vi "Load Class.vi"(8 "error in":errorcluster, 10 "PPLs Folder Path":path, 11 "Configuration in":refnum<class "Configuration.lvclass">) -> (0 "error out":errorcluster, 2 "Class out":refnum<class>, 3 "Configuration out":refnum<class "Configuration.lvclass">)   [LabVIEW 2018, in "Configuration.lvlib" / "Configuration.lvclass"]
doc: "Load the specific class and return a generic class instantiation"
uses:
  Configuration.lvclass
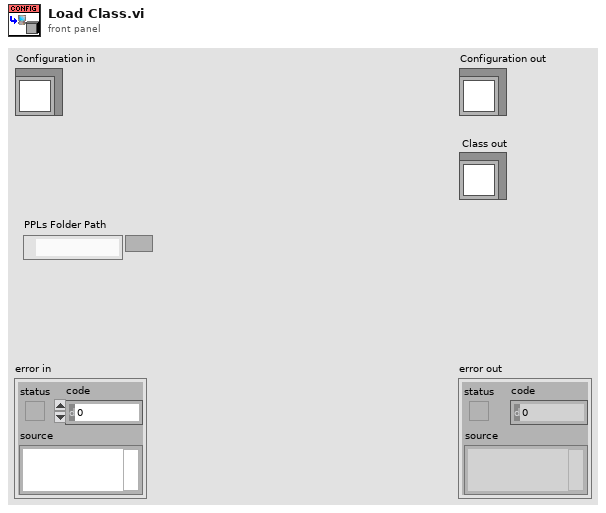
[diagram p1: front panel]
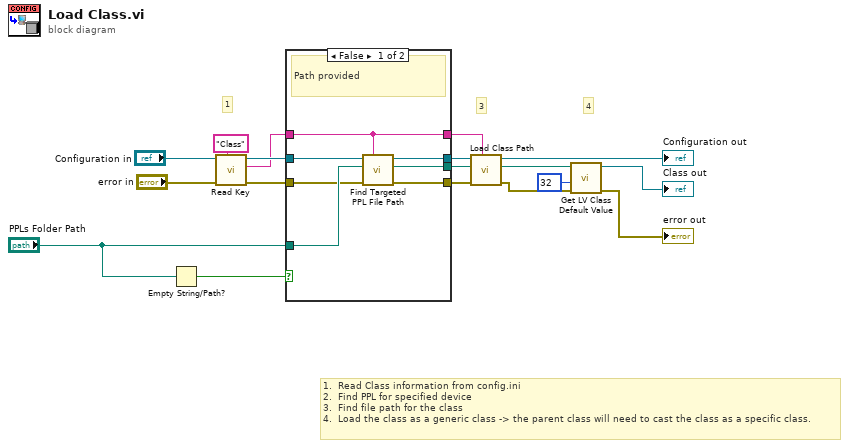
[diagram p0: block diagram]
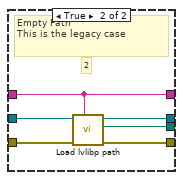
[diagram p2: hidden frame]
diagram:
  # "1.  Read Class information from config.ini\n2.  Find PPL for specified device\n3.  Find file path for the class\n4.  Load the class as a generic class -> the parent class will need to cast the class as a specific class."
  # "4"
  # "3"
  # "1"
  n1 = Empty String/Path?(string/path="PPLs Folder Path") -> (empty?=w2:bool)
  n2 = call "Read Key.vi"("Key:"="Class", "error in"="error in", "Configuration in"="Configuration in") -> ("error out"=w12:errorcluster, "Value"=w10:string, "Configuration out"=w11:refnum<class "Configuration.lvclass">)  [unwired: 6 in]
  n3 = case shown="False" w2 {
    tunnel: [w19 w31] -> w15
    tunnel: [w20 w30] -> w14
    tunnel: [w21 w29] -> w13
    tunnel: w12 -> [w23 w28]
    tunnel: w11 -> [w25 w27]
    tunnel: w10 -> [w22 w26]
    tunnel: [w22 w26] -> w3
    tunnel: "PPLs Folder Path" -> [w24 _]
    frame False {
      # "Path provided"
      n4 = call "Find Targeted PPL File Path.vi"("error in (no error)"=w23, "Class Name"=w22, "PPLs Folder Path"=w24, "Configuration in"=w25) -> ("error out"=w20:errorcluster, "PPL File Path"=w19:path, "Configuration out"=w21:refnum<class "Configuration.lvclass">)  [unwired: 5 in]
    }
    frame True {
      # "2"
      # "Empty Path\nThis is the legacy case"
      n5 = call "Load lvlibp path.vi"("Class Name"=w26, "error in"=w28, "Configuration in"=w27) -> ("error out"=w30:errorcluster, "lvlibp Path"=w31:path, "Configuration out"=w29:refnum<class "Configuration.lvclass">)  [unwired: 6 in]
    }
  }
  n6 = call "Load Class Path.vi"("Class Name"=w3, "error in"=w14, "lvlibp path"=w15, "Configuration in"=w13) -> ("error out"=w8:errorcluster, "Class Path"=w9:path, "Configuration out"=→"Configuration out":refnum<class "Configuration.lvclass">)  [unwired: 5 in]
  n7 = call <vilib>:"Get LV Class Default Value.vi"("error in (no error)"=w8, "options"=u32 32, "class path"=w9) -> ("error out"=→"error out":errorcluster, "object"=→"Class out":refnum<class>)  [unwired: 7 in]
